vi "FactorCorreccion.vi"(8 "error in (no error)":errorcluster, 10 "Nivel Medido":dbl format="%#.2g", 11 "Nivel Emitido":dbl) -> (0 "error out":errorcluster, 3 "factor_correccion":dbl format="%#.5g")   [LabVIEW 2019, in "AjustesPrevios.lvclass"]
uses:
  AjustesPrevios.lvclass
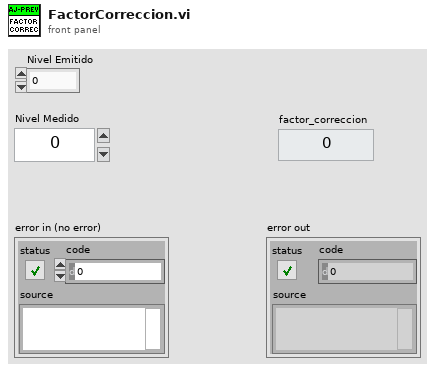
[diagram p1: front panel]
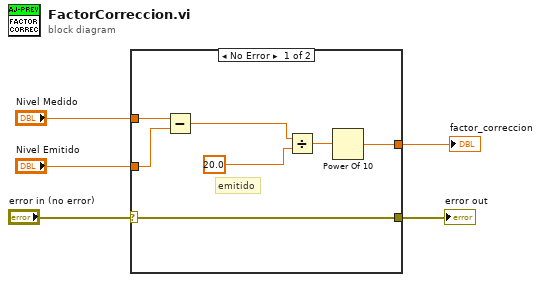
[diagram p0: block diagram]
diagram:
  n1 = case shown="No Error" "error in (no error)" {
    selector: "error in (no error)" -> [w6 w13]
    tunnel: [w12 _] -> w5
    tunnel: "Nivel Medido" -> [w9 _]
    tunnel: "Nivel Emitido" -> [w8 _]
    tunnel: [w6 w13] -> w1
    frame No Error {
      # "emitido"
      n2 = Subtract(x=w9, y=w8) -> (x-y=w7:dbl)
      n3 = Divide(x=w7, y=20.0) -> (x/y=w10:dbl)
      n4 = Power Of 10(x=w10) -> (10^x=w12:dbl)
    }
    frame Error {
    }
  }
  "factor_correccion" <- w5
  "error out" <- w1
